vi "SwissSPAD Live_Compute SS2 Gate Characteristics.vi"(7 "Gate Characteristics Refnum":refnum<vi>, 8 "Error In":errorcluster, 11 "SS2 DAQ Parameters":T2={"10 bits"=FALSE, "# Exposure Sequences"=0, "# 1-bit Frame per Gate"=255, "Gate Shift"=0, "# Gates per Set"=0, "# Sets"=1, "Laser Period"=0.0, "Sync Period"=0.0, "Gate Offset"=0, "Auto-adjust Gate Offset"=FALSE, "Gate Definition"={"gs_psincdec_0"=0, "gs_psincdec_1"=0, "gs_psincdec_2"=0, "gs_psincdec_3"=0, "gs_no_shift_adj_1"=0, "gs_no_shift_adj_2"=0, "gs_no_shift_adj_3"=0}, "Reversed Shift"=FALSE} {"Sync Period" min=0.0 max=4.294967295; "# Sets" min=1}) -> (0 "Error Out":errorcluster, 3 "Gate Characteristics":T1)   [LabVIEW 2021]
uses:
  SwissSPAD Live_SS2 DAQ Parameters 3.ctl
  SwissSPAD Live_SS2 Gate Definition.ctl
  SwissSPAD Live_Gate Characteristics.ctl
panel:
  out "Delta Recharge/Gate":dbl
  out "Recharge Duration":dbl
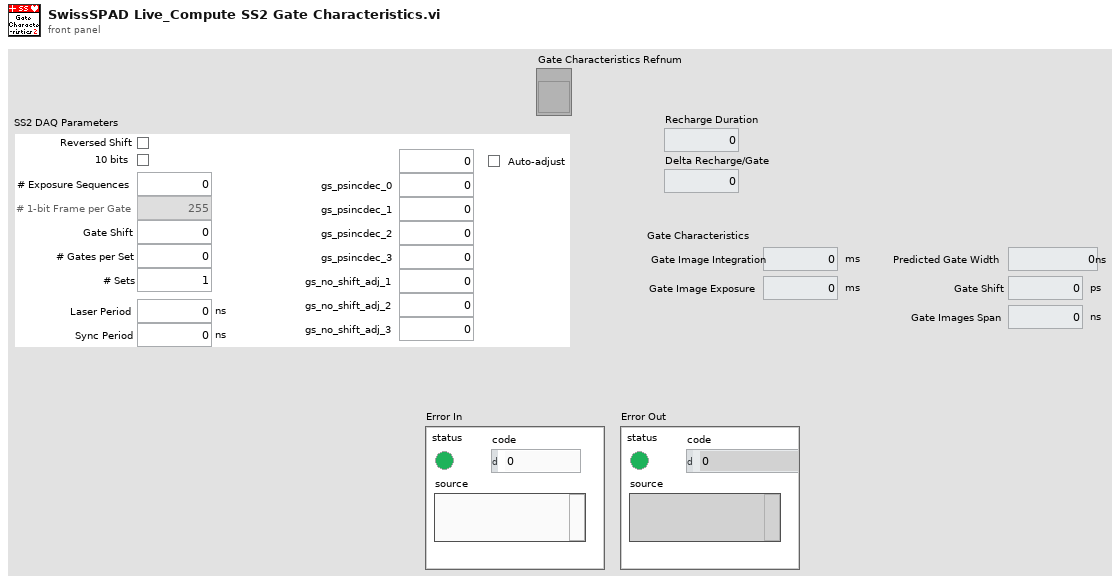
[diagram p1: front panel]
types:
  T1 = typedef "SwissSPAD Live_Gate Characteristics.ctl" = cluster{"Predicted Gate Width":dbl[unit], "Gate Image Integration":dbl[unit], "Gate Image Exposure":dbl[unit], "Gate Shift":dbl[unit], "Gate Images Span":dbl[unit]}
  T2 = typedef "SwissSPAD Live_SS2 DAQ Parameters 3.ctl" = cluster{"10 bits":bool, "# Exposure Sequences":u32, "# 1-bit Frame per Gate":u32, "Gate Shift":u32, "# Gates per Set":u32, "# Sets":u32, "Laser Period":dbl[unit], "Sync Period":dbl[unit], "Gate Offset":u32, "Auto-adjust Gate Offset":bool, "Gate Definition":T3, "Reversed Shift":bool}
  T3 = typedef "SwissSPAD Live_SS2 Gate Definition.ctl" = cluster{"gs_psincdec_0":u32, "gs_psincdec_1":u32, "gs_psincdec_2":u32, "gs_psincdec_3":u32, "gs_no_shift_adj_1":u32, "gs_no_shift_adj_2":u32, "gs_no_shift_adj_3":u32}
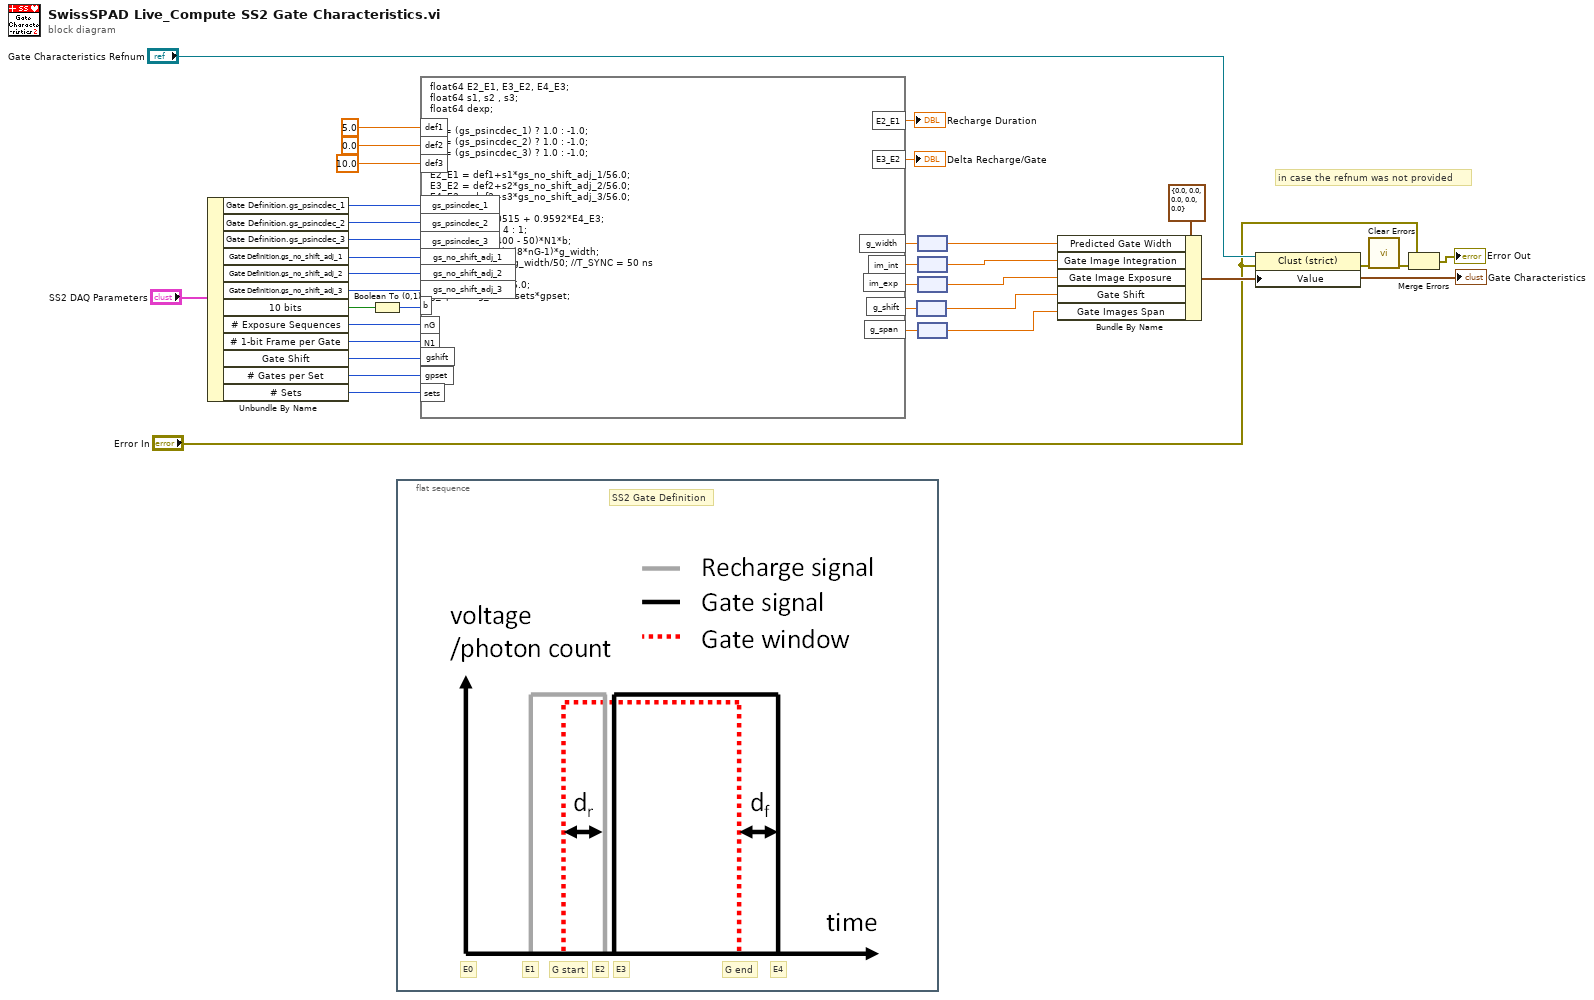
[diagram p0: block diagram]
diagram:
  # "in case the refnum was not provided"
  n1 = Unbundle By Name("SS2 DAQ Parameters") -> ("Gate Definition.gs_psincdec_1"=w33:u32, "Gate Definition.gs_psincdec_2"=w32:u32, "Gate Definition.gs_psincdec_3"=w31:u32, "Gate Definition.gs_no_shift_adj_1"=w30:u32, "Gate Definition.gs_no_shift_adj_2"=w29:u32, "Gate Definition.gs_no_shift_adj_3"=w28:u32, "10 bits"=w23:bool, "# Exposure Sequences"=w21:u32, "# 1-bit Frame per Gate"=w20:u32, "Gate Shift"=w13:u32, "# Gates per Set"=w8:u32, "# Sets"=w7:u32)
  n2 = Boolean To (0,1)(Boolean=w23) -> (0, 1=w22:i16)
  n3 = flat-sequence {
    frame #0 {
      # "SS2 Gate Definition"
      # "G end"
      # "G start"
      # "E0"
      # "E4"
      # "E3"
      # "E2"
      # "E1"
    }
  }
  n4 = formula code="float64 E2_E1, E3_E2, E4_E3;\nfloat64 s1, s2 , s3;\nfloat64 dexp;\n\ns1 = (gs_psincdec_1) ? 1.0 : -1.0; \ns2 = (gs_psincdec_2) ? 1.0 : -1.0; \ns3 = (gs_psincdec_3) ? 1.0 : -1.0; \n\nE2_E1 = def1+s1*gs_no_shift_adj_1/56.0;\nE3_E2 = def2+s2*gs_no_shift_adj_2/56.0;\nE4_E3 = def3+s3*gs_no_shift_adj_3/56.0;\n\ng_width = 2.60515 + 0.9592*E4_E3;\nb = (b == 1) ? 4 : 1;\nim_int = (nG*400 - 50)*N1*b;\n//im_exp = N1*b*(8*nG-1)*g_width;\nim_exp = im_int*g_width/50; //T_SYNC = 50 ns\n\ng_shift = gshift/56.0;\ng_span = g_shift*sets*gpset;"("def1"=5.0 ("input variable"), "def2"=0.0 ("input variable"), "def3"=10.0 ("input variable"), "gs_psincdec_1"=w33, "gs_psincdec_2"=w32, "gs_psincdec_3"=w31, "gs_no_shift_adj_1"=w30, "gs_no_shift_adj_2"=w29, "gs_no_shift_adj_3"=w28, "b"=w22, "nG"=w21, "N1"=w20, "gshift"=w13, "gpset"=w8, "sets"=w7) -> ("g_width"=w27:dbl, "E2_E1"=→"Recharge Duration":dbl, "E3_E2"=→"Delta Recharge/Gate":dbl, "im_int"=w19:dbl, "im_exp"=w18:dbl, "g_shift"=w12:dbl, "g_span"=w10:dbl)
  n5 = node(w12) -> (w11:dbl[unit])
  n6 = node(w27) -> (w16:dbl[unit])
  n7 = node(w19) -> (w15:dbl[unit])
  n8 = node(w18) -> (w14:dbl[unit])
  n9 = node(w10) -> (w9:dbl[unit])
  n10 = Bundle By Name(cluster=T1 {"Predicted Gate Width"=0.0, "Gate Image Integration"=0.0, "Gate Image Exposure"=0.0, "Gate Shift"=0.0, "Gate Images Span"=0.0} ("Gate Characteristics"), "Predicted Gate Width"=w16, "Gate Image Integration"=w15, "Gate Image Exposure"=w14, "Gate Shift"=w11, "Gate Images Span"=w9) -> (w4:T1)
  "Gate Characteristics" <- w4
  n11 = property class="Clust (strict)"(reference="Gate Characteristics Refnum", error in="Error In", "Value"=w4) -> (error out=w5:errorcluster)  [unwired: 1 out]
  n12 = call <vilib>:"Clear Errors.vi"("error in (no error)"=w5) -> ("error out"=w3:errorcluster)  [unwired: 5 in, 1 out]
  n13 = Merge Errors("Error In", w3) -> (→"Error Out":errorcluster)
